vi "config.vi"(5 "Function":enum16{"write", "read"}(ring), 6 "Error In":errorcluster, 7 "Instrument":T3(ring), 8 "Amplifiers":enum16{"None", "Krohn Hite", "Femto"}(ring), 9 "DAQ Type":enum16{"None", "USB 4431", "PXI 446x"}(ring), 10 "AO Configuration":T1(array[cluster])=[{"Output physical channels"="PXI1Slot2/ao0:1", "AO. Max"=1.0, "AO.Min"=-1.0}, {"Output physical channels"="PXI1Slot3/ao0:1", "AO. Max"=1.0, "AO.Min"=-1.0}, {"Output physical channels"="PXI1Slot5/ao0:1", "AO. Max"=1.0, "AO.Min"=-1.0}], 11 "AI Configuration":T2(array[cluster])=[{"AI.Coupling"=enum."GND", "AI.Max"=1.0, "AI.Min"=-1.0, "Input physical channels"="PXI1Slot2/ai0:1"}, {"AI.Coupling"=enum."GND", "AI.Max"=1.0, "AI.Min"=-1.0, "Input physical channels"="PXI1Slot3/ai0:1"}, {"AI.Coupling"=enum."GND", "AI.Max"=1.0, "AI.Min"=-1.0, "Input physical channels"="PXI1Slot5/ai0:1"}]) -> (0 "Amplifiers":enum16{"None", "Krohn Hite", "Femto"}(ring), 1 "DAQ Type":enum16{"None", "USB 4431", "PXI 446x"}(ring), 2 "AO Configuration 2":T1(array[cluster])=[{"Output physical channels"="PXI1Slot2/ao0:1", "AO. Max"=1.0, "AO.Min"=-1.0}, {"Output physical channels"="PXI1Slot3/ao0:1", "AO. Max"=1.0, "AO.Min"=-1.0}, {"Output physical channels"="PXI1Slot5/ao0:1", "AO. Max"=1.0, "AO.Min"=-1.0}], 3 "AI Configuration 2":T2(array[cluster])=[{"AI.Coupling"=enum."GND", "AI.Max"=1.0, "AI.Min"=-1.0, "Input physical channels"="PXI1Slot2/ai0:1"}, {"AI.Coupling"=enum."GND", "AI.Max"=1.0, "AI.Min"=-1.0, "Input physical channels"="PXI1Slot3/ai0:1"}, {"AI.Coupling"=enum."GND", "AI.Max"=1.0, "AI.Min"=-1.0, "Input physical channels"="PXI1Slot5/ai0:1"}], 4 "Error Out":errorcluster)   [LabVIEW 2013]
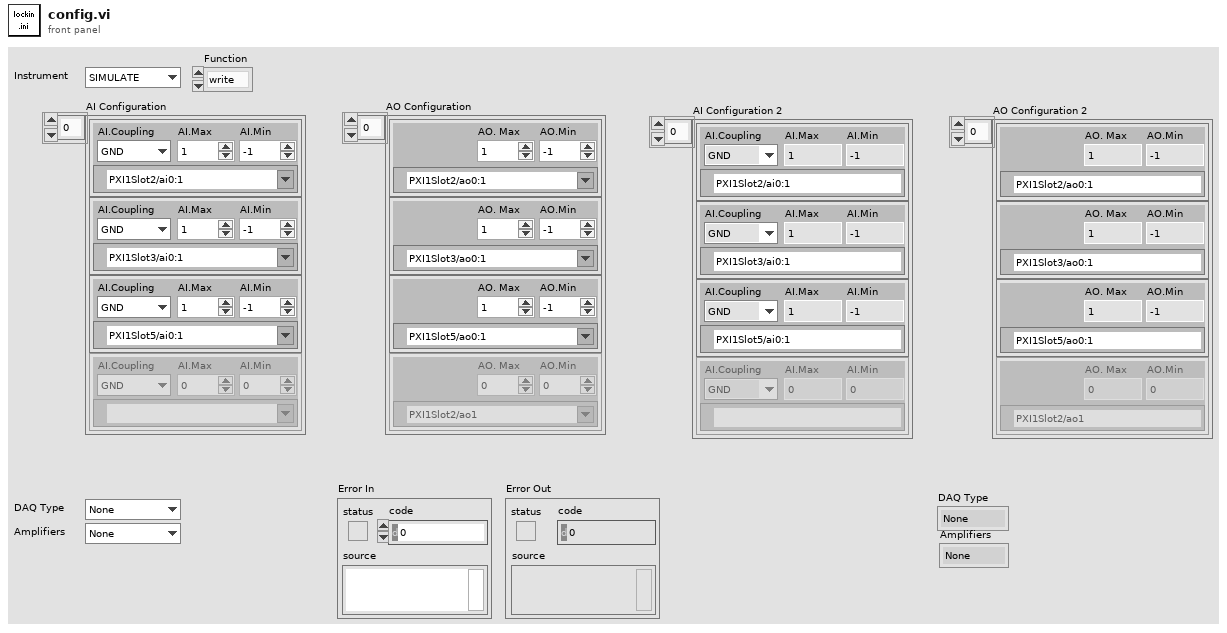
[diagram p1: front panel]
types:
  T1 = cluster{"Output physical channels":tag, "AO. Max":dbl, "AO.Min":dbl}[]
  T2 = cluster{"AI.Coupling":enum16{"AC", "DC", "GND"}, "AI.Max":dbl, "AI.Min":dbl, "Input physical channels":tag}[]
  T3 = enum16{"SIMULATE", "CF900", "DR200", "MNK", "PPMS1", "PPMS2", "THz1", "THz2"}
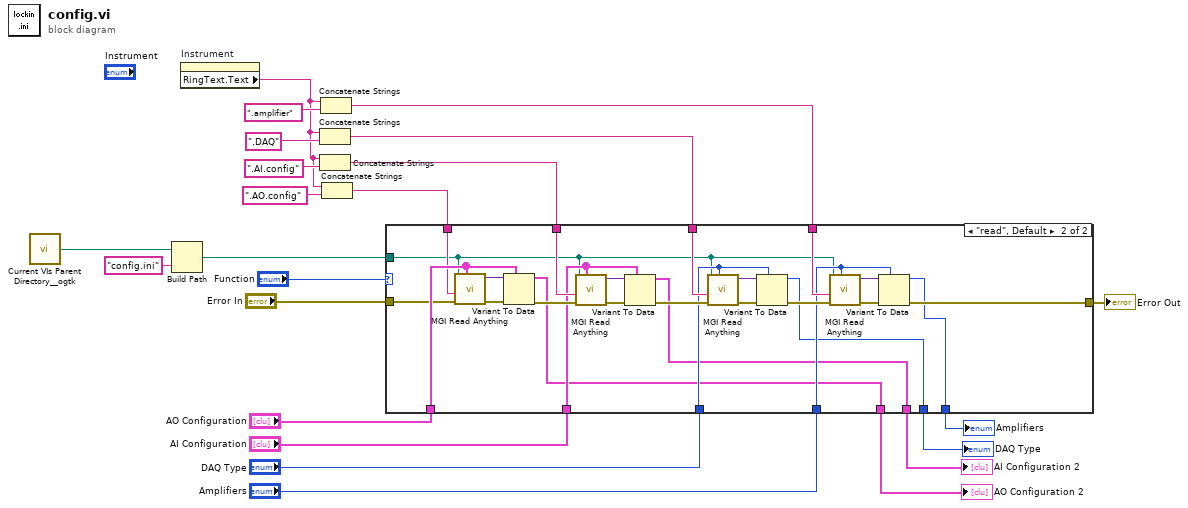
[diagram p0: block diagram]
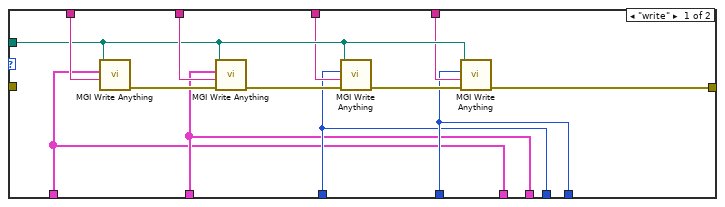
[diagram p2: hidden frame]
diagram:
  n1 = call <userlib>:"Current VIs Parent Directory__ogtk.vi"() -> ("Parent Directory (+ Relative)"=w23:path)  [unwired: 5 in]
  n2 = Build Path(base path=w23, name or relative path="config.ini") -> (appended path=w17:path)
  n3 = property on="Instrument" class="Enum (strict)"() -> ("RingText.Text"=w11:string)  [unwired: 2 in, 2 out]
  n4 = Concatenate Strings(w11, ".DAQ" ("Section Name (Name of \"Anything\")")) -> (w8:string)
  n5 = Concatenate Strings(w11, ".AI.config" ("Section Name (Name of \"Anything\")")) -> (w9:string)
  n6 = Concatenate Strings(w11, ".amplifier" ("Section Name (Name of \"Anything\")")) -> (w7:string)
  n7 = Concatenate Strings(w11, ".AO.config" ("Section Name (Name of \"Anything\")")) -> (w10:string)
  n8 = case shown="\"read\", Default" "Function" {
    tunnel: w10 -> [w36 w53]
    tunnel: "AI Configuration" -> [w25 w47]
    tunnel: w9 -> [w34 w52]
    tunnel: "AO Configuration" -> [w24 w60]
    tunnel: "DAQ Type" -> [w26 w46]
    tunnel: "Amplifiers" -> [w27 w44]
    tunnel: w17 -> [w31 w41]
    tunnel: [w30 w43] -> w16
    tunnel: w8 -> [w29 w51]
    tunnel: w7 -> [w28 w50]
    tunnel: "Error In" -> [_ w42]
    tunnel: [w24 w40] -> w4
    tunnel: [w25 w39] -> w3
    tunnel: [w26 w38] -> w2
    tunnel: [w27 w37] -> w1
    frame "write" {
      n9 = call <userlib>:"MGI Write Anything.vi"("Section Name (Name of \"Anything\")"=w36, "Anything"=w24, "Path (dialog)"=w31) -> ("Error Out"=w35:errorcluster)  [unwired: 6 in, 2 out]
      n10 = call <userlib>:"MGI Write Anything.vi"("Error In"=w35, "Section Name (Name of \"Anything\")"=w34, "Anything"=w25, "Path (dialog)"=w31) -> ("Error Out"=w33:errorcluster)  [unwired: 5 in, 2 out]
      n11 = call <userlib>:"MGI Write Anything.vi"("Error In"=w33, "Section Name (Name of \"Anything\")"=w29, "Anything"=w26, "Path (dialog)"=w31) -> ("Error Out"=w32:errorcluster)  [unwired: 5 in, 2 out]
      n12 = call <userlib>:"MGI Write Anything.vi"("Error In"=w32, "Section Name (Name of \"Anything\")"=w28, "Anything"=w27, "Path (dialog)"=w31) -> ("Error Out"=w30:errorcluster)  [unwired: 5 in, 2 out]
    }
    frame "read", Default {
      n13 = call <userlib>:"MGI Read Anything.vi"("Type of Anything"=w60, "Error In"=w42, "Section Name (Name of \"Type of Anything\")"=w53, "Path (dialog)"=w41) -> ("Error Out"=w62:errorcluster, "Anything"=w61:variant)  [unwired: 4 in, 2 out]
      n14 = Variant To Data(error in=w62, type=w60, Variant=w61) -> (data=w40:T1, error out=w58:errorcluster)
      n15 = call <userlib>:"MGI Read Anything.vi"("Type of Anything"=w47, "Error In"=w58, "Section Name (Name of \"Type of Anything\")"=w52, "Path (dialog)"=w41) -> ("Error Out"=w59:errorcluster, "Anything"=w48:variant)  [unwired: 4 in, 2 out]
      n16 = Variant To Data(error in=w59, type=w47, Variant=w48) -> (data=w39:T2, error out=w56:errorcluster)
      n17 = call <userlib>:"MGI Read Anything.vi"("Type of Anything"=w46, "Error In"=w56, "Section Name (Name of \"Type of Anything\")"=w51, "Path (dialog)"=w41) -> ("Error Out"=w57:errorcluster, "Anything"=w49:variant)  [unwired: 4 in, 2 out]
      n18 = Variant To Data(error in=w57, type=w46, Variant=w49) -> (data=w38:enum16{"None", "USB 4431", "PXI 446x"}, error out=w54:errorcluster)
      n19 = call <userlib>:"MGI Read Anything.vi"("Type of Anything"=w44, "Error In"=w54, "Section Name (Name of \"Type of Anything\")"=w50, "Path (dialog)"=w41) -> ("Error Out"=w55:errorcluster, "Anything"=w45:variant)  [unwired: 4 in, 2 out]
      n20 = Variant To Data(error in=w55, type=w44, Variant=w45) -> (data=w37:enum16{"None", "Krohn Hite", "Femto"}, error out=w43:errorcluster)
    }
  }
  "Error Out" <- w16
  "AO Configuration 2" <- w4
  "AI Configuration 2" <- w3
  "DAQ Type" <- w2
  "Amplifiers" <- w1
